vi "Log Message to File.vi"(8 "error in (no error)":errorcluster, 10 "Message Data":string[](array[string]), 11 "Message Log in":refnum<class "Message Log.lvclass">) -> (0 "error out":errorcluster, 3 "Message Log out":refnum<class "Message Log.lvclass">)   [LabVIEW 2017, in "Message Log.lvclass"]
uses:
  Message Log.lvclass
  Message Log.lvclass/Message Log.ctl
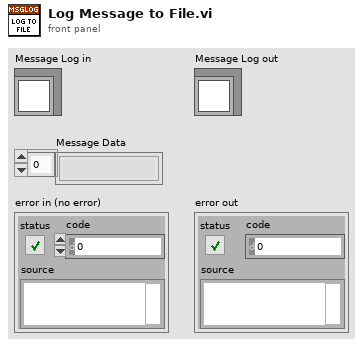
[diagram p1: front panel]
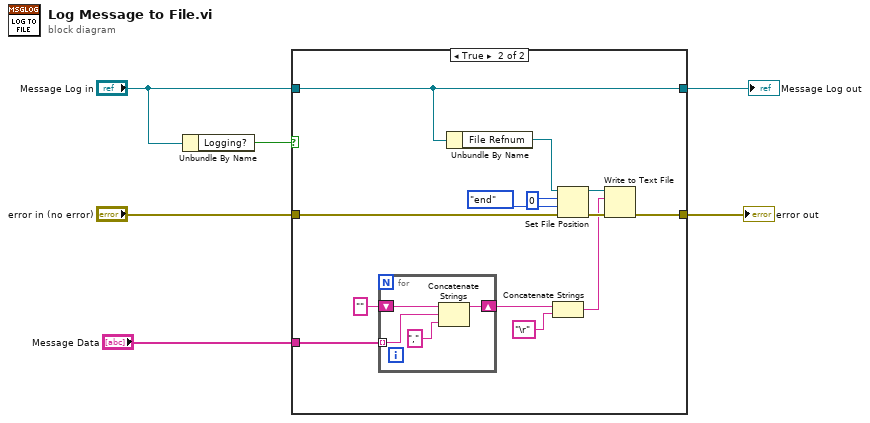
[diagram p0: block diagram]
diagram:
  n1 = Unbundle By Name("Message Log in") -> ("Logging?"=w5:bool)
  n2 = case shown="True" w5 {
    tunnel: "Message Data" -> [_ w18]
    tunnel: "Message Log in" -> [w8 w9]
    tunnel: "error in (no error)" -> [w7 w11]
    tunnel: [w7 w10] -> w2
    tunnel: [w8 w9] -> w3
    frame False {
    }
    frame True {
      n3 = for {
        tunnel: w18 -> [w23] mode=indexing
        shift-right: [w24] -> w20
        shift-left: "" -> [w25]
        n4 = Concatenate Strings(w25, w23, "," ("string")) -> (w24:string)
      }
      n5 = Unbundle By Name(w9) -> ("File Refnum"=w12:refnum<file>)
      n6 = Concatenate Strings(w20, "\r" ("string")) -> (w13:string)
      n7 = Set File Position(offset (in bytes) (0)=i64 0, refnum=w12, from (0:start)=enum16{"start", "end", "current"}."end", error in=w11) -> (refnum out=w14:refnum<file>, error out=w15:errorcluster)
      n8 = Write to Text File(file (use dialog)=w14, text=w13, error in=w15) -> (error out=w10:errorcluster)  [unwired: 1 in, 2 out]
    }
  }
  "Message Log out" <- w3
  "error out" <- w2
